vi "Destroy Events.vi"(8 "error in (no error)":errorcluster, 11 "Guardian in":refnum<class "Guardian.lvclass">) -> (0 "error out":errorcluster, 3 "Guardian out":refnum<class "Guardian.lvclass">)   [LabVIEW 2026, in "TALOS.lvlib" / "Guardian.lvlib" / "Guardian.lvclass"]
uses:
  Guardian.lvclass
  C:/LabVIEW Code/TALOS/talos/Ancestor/Ancestor/Ancestor.lvclass
  <vilib>/event_ctls.llb/usereventprio.ctl
  Guardian.lvclass/Guardian.ctl
  Classes/uService List/uService List.lvclass
  Classes/Error Filter/Error Filter.lvclass
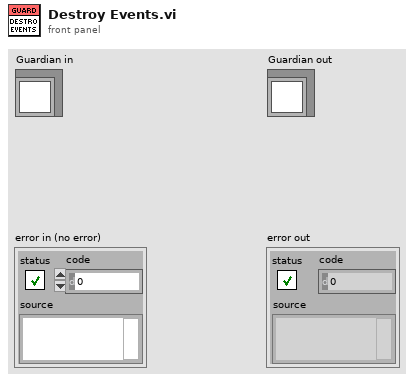
[diagram p1: front panel]
types:
  T1 = typedef "usereventprio.ctl" = enum32{"high priority", "normal priority"}
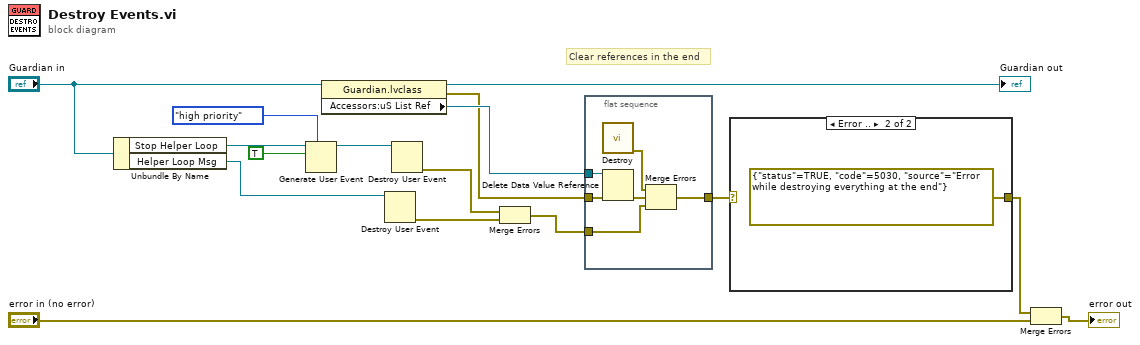
[diagram p0: block diagram]
diagram:
  # "Clear references in the end"
  n1 = Unbundle By Name("Guardian in") -> ("Stop Helper Loop"=w16:refnum<user-event>, "Helper Loop Msg"=w6:refnum<user-event>)
  n2 = Generate User Event(priority (normal)=usereventprio."high priority", user event=w16, event data cluster=TRUE ("event data")) -> (user event out=w13:refnum<user-event>)  [unwired: 1 in, 1 out]
  n3 = property class="Guardian.lvclass"(reference="Guardian in") -> (reference out=→"Guardian out":refnum<class "Guardian.lvclass">, error out=w8:errorcluster, "Accessors:uS List Ref"=w9:refnum<data-value>)  [unwired: 1 in]
  n4 = Destroy User Event(user event=w6) -> (error out=w5:errorcluster)  [unwired: 1 in]
  n5 = Destroy User Event(user event=w13) -> (error out=w11:errorcluster)  [unwired: 1 in]
  n6 = Merge Errors(w11, w5) -> (w7:errorcluster)
  n7 = flat-sequence {
    tunnel: w9 -> [w22]
    tunnel: w8 -> [w21]
    tunnel: [w19] -> w4
    tunnel: w7 -> [w18]
    frame #0 {
      n8 = call "Destroy.vi"() -> ("error out"=w17:errorcluster)  [unwired: 11 in]
      n9 = Delete Data Value Reference(data value reference=w22, error in=w21) -> (error out=w20:errorcluster)  [unwired: 1 out]
      n10 = Merge Errors(w17, w20, w18) -> (w19:errorcluster)
    }
  }
  n11 = case shown="Error .." w4 {
    selector: w4 -> [w23 _]
    tunnel: [w23 errorcluster {"status"=TRUE, "code"=5030, "source"="Error while destroying everything at the end"} ("error IO")] -> w3
    frame No Error {
    }
    frame Error {
    }
  }
  n12 = Merge Errors(w3, "error in (no error)") -> (→"error out":errorcluster)
